vi "Script Work CS.vi"(6 "State":T1={"Worker Library Path"=path "", "Block Label"="", "Types"=[], "Selections"=[], "Icon"={"image type"=0, "image depth"=0, "image"=[], "mask"=[], "colors"=[], "Rectangle"={"left"=0, "top"=0, "right"=0, "bottom"=0}}, "Errors"={"Terminals"=[], "Generate"={"status"=FALSE, "code"=0, "source"=""}, "General"={"status"=FALSE, "code"=0, "source"=""}}, "Calculated Sizes"={"Block Width"=0, "Block Height"=0, "Half Width"=0, "Icon Top"=0, "Icon Bottom"=0, "Label Width"=0, "Half Label"=0, "Label Top"=0, "Text Width"=0, "Half Text"=0, "Text Height"=0, "Label Height"=0, "Expanded Width"=0, "Label Bottom"=0, "Expanded Top"=0, "Expanded Bottom"=0, "Expanded Height"=0, "Min Height"=0, "Max Height"=0}, "Special Terminal Indices"={"Action"=-1, "Init"=-1, "Tag"=-1, "State in"=-1, "State out"=-1, "Error"=-1, "Control"=-1}, "Terminals"=[]}, 8 "error in (no error)":errorcluster, 11 "Refs In":T13) -> (0 "error out":errorcluster, 3 "Refs":T13)   [LabVIEW 2022 SP3, in "FlexBlocks Support.lvlib"]
uses:
  FlexBlocks Support.lvlib
  SM Refs.ctl
  Flex Block/State.ctl
  Type Descriptor.ctl
  Terminal Direction.ctl
  Value Mode.ctl
  Special Terminal.ctl
  <vilib>/picture/picture.llb/imagedata.ctl
  XNode Errors.ctl
  Calculated Sizes.ctl
  Special Terminal Indices.ctl
  Terminal Status.ctl
  Terminal State.ctl
  Terminal Draw Style.ctl
  Flex Block/Flex Block.xnode
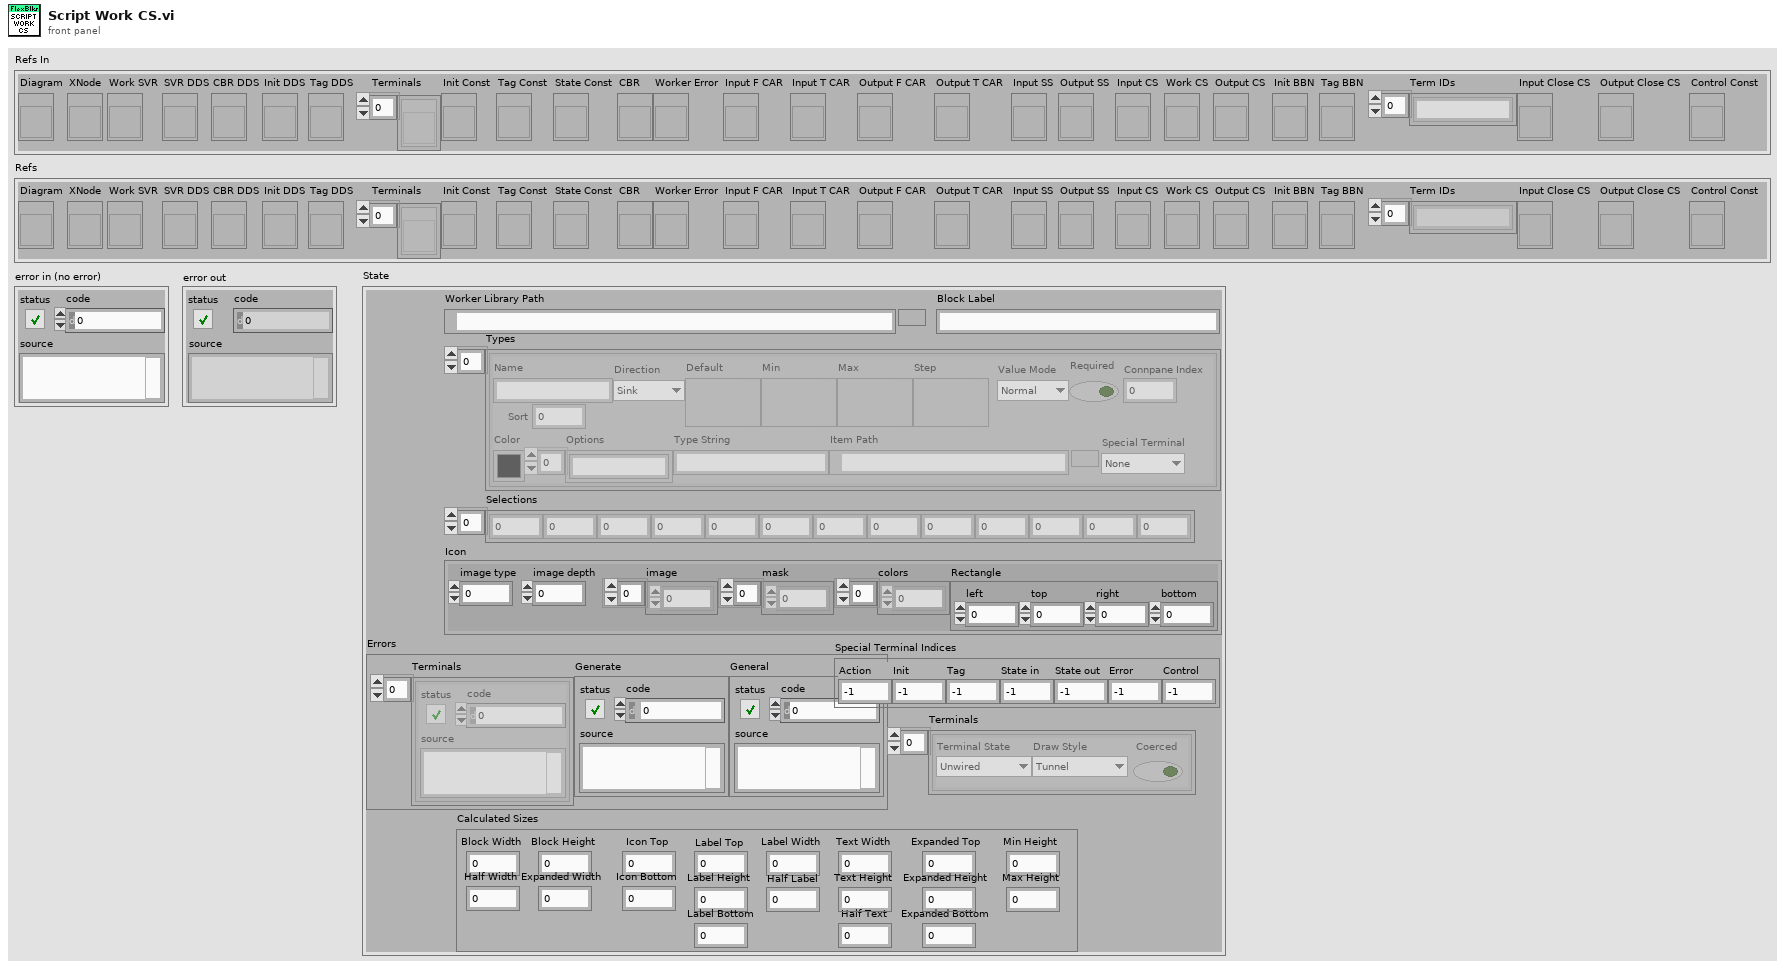
[diagram p1: front panel]
types:
  T1 = typedef "Flex Block.xnode/State.ctl" = cluster{"Worker Library Path":path, "Block Label":string, "Types":T2[], "Selections":i32[], "Icon":T6, "Errors":T7, "Calculated Sizes":T8, "Special Terminal Indices":T9, "Terminals":T10[]}
  T2 = typedef "FlexBlocks Support.lvlib/Type Descriptor.ctl" = cluster{"Name":string, "Direction":T3, "Default":variant, "Min":variant, "Max":variant, "Step":variant, "Value Mode":T4, "Color":u32, "Options":string[], "Type String":string, "Item Path":path, "Required":bool, "Connpane Index":i32, "Special Terminal":T5, "Sort":i32}
  T3 = typedef "FlexBlocks Support.lvlib/Terminal Direction.ctl" = enum16{"Sink", "Source"}
  T4 = typedef "FlexBlocks Support.lvlib/Value Mode.ctl" = enum16{"Normal", "Range", "Select"}
  T5 = typedef "FlexBlocks Support.lvlib/Special Terminal.ctl" = enum16{"None", "Action", "Init", "Tag", "State in", "State out", "Error", "Control"}
  T6 = typedef "imagedata.ctl" = cluster{"image type":i32, "image depth":i32, "image":u8[], "mask":u8[], "colors":u32[], "Rectangle":cluster{"left":i16, "top":i16, "right":i16, "bottom":i16}}
  T7 = typedef "FlexBlocks Support.lvlib/XNode Errors.ctl" = cluster{"Terminals":errorcluster[], "Generate":errorcluster, "General":errorcluster}
  T8 = typedef "FlexBlocks Support.lvlib/Calculated Sizes.ctl" = cluster{"Block Width":i32, "Block Height":i32, "Half Width":i32, "Icon Top":i32, "Icon Bottom":i32, "Label Width":i32, "Half Label":i32, "Label Top":i32, "Text Width":i32, "Half Text":i32, "Text Height":i32, "Label Height":i32, "Expanded Width":i32, "Label Bottom":i32, "Expanded Top":i32, "Expanded Bottom":i32, "Expanded Height":i32, "Min Height":i32, "Max Height":i32}
  T9 = typedef "FlexBlocks Support.lvlib/Special Terminal Indices.ctl" = cluster{"Action":i32, "Init":i32, "Tag":i32, "State in":i32, "State out":i32, "Error":i32, "Control":i32}
  T10 = typedef "FlexBlocks Support.lvlib/Terminal Status.ctl" = cluster{"Terminal State":T11, "Draw Style":T12, "Coerced":bool}
  T11 = typedef "FlexBlocks Support.lvlib/Terminal State.ctl" = enum16{"Unwired", "BadType", "BadRef", "Channel", "Value", "Control Ref"}
  T12 = typedef "FlexBlocks Support.lvlib/Terminal Draw Style.ctl" = enum16{"Tunnel", "BadType", "BadRef", "Channel", "Value", "Control Ref"}
  T13 = typedef "FlexBlocks Support.lvlib/SM Refs.ctl" = cluster{"Diagram":refnum<vi>, "XNode":refnum<vi>, "Work SVR":refnum<vi>, "SVR DDS":refnum<vi>, "CBR DDS":refnum<vi>, "Init DDS":refnum<vi>, "Tag DDS":refnum<vi>, "Terminals":refnum<vi>[], "Init Const":refnum<vi>, "Tag Const":refnum<vi>, "State Const":refnum<vi>, "CBR":refnum<vi>, "Worker Error":refnum<vi>, "Input F CAR":refnum<vi>, "Input T CAR":refnum<vi>, "Output F CAR":refnum<vi>, "Output T CAR":refnum<vi>, "Input SS":refnum<vi>, "Output SS":refnum<vi>, "Input CS":refnum<vi>, "Work CS":refnum<vi>, "Output CS":refnum<vi>, "Init BBN":refnum<vi>, "Tag BBN":refnum<vi>, "Term IDs":string[], "Input Close CS":refnum<vi>, "Output Close CS":refnum<vi>, "Control Const":refnum<vi>}
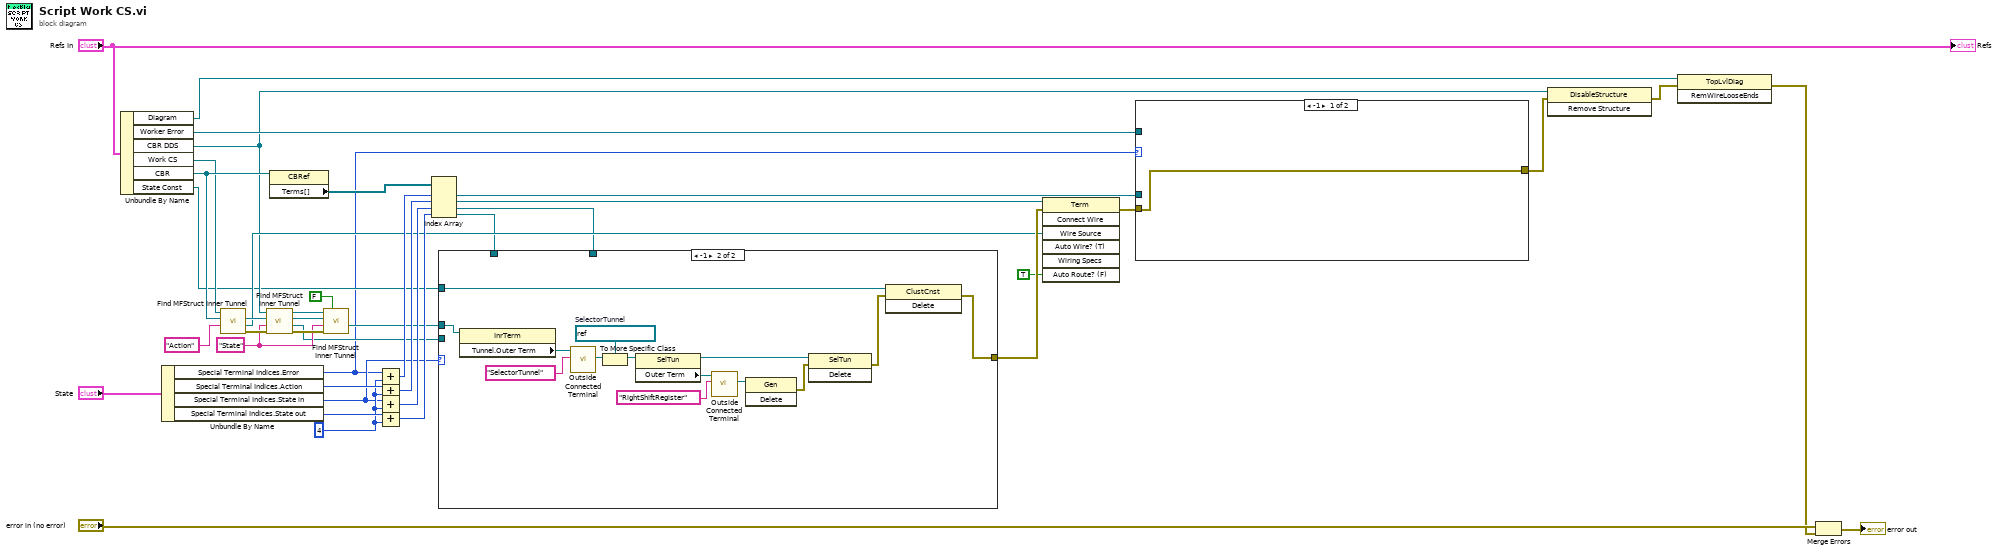
[diagram p0: block diagram]
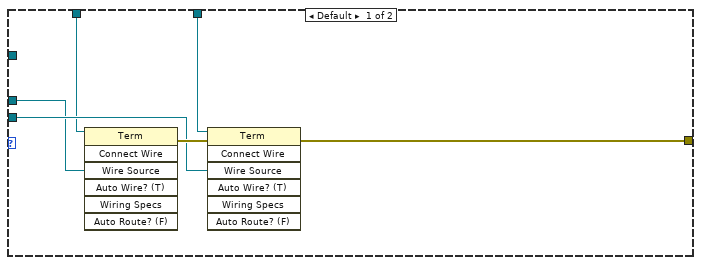
[diagram p2: hidden frame]
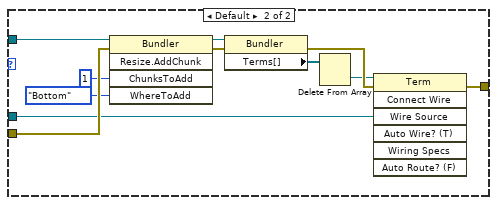
[diagram p3: hidden frame]
diagram:
  w27 = 4 ("y")
  w35 = "State" ("Tunnel Name")
  n1 = Unbundle By Name("Refs In") -> ("Diagram"=w5:refnum<vi>, "Worker Error"=w18:refnum<vi>, "CBR DDS"=w13:refnum<vi>, "Work CS"=w12:refnum<vi>, "CBR"=w20:refnum<vi>, "State Const"=w4:refnum<vi>)
  n2 = Unbundle By Name("State") -> ("Special Terminal Indices.Error"=w1:i32, "Special Terminal Indices.Action"=w28:i32, "Special Terminal Indices.State in"=w11:i32, "Special Terminal Indices.State out"=w31:i32)
  n3 = call "Find MFStruct Inner Tunnel.vi"("Tunnel Name"="Action", "Contained GObject"=w20, "MFStruct"=w12) -> ("error IO"=w39:errorcluster, "Inside Tunnel"=w19:refnum<vi>, "GObject dup"=w22:refnum<vi>)  [unwired: 5 in, 1 out]
  n4 = call "Find MFStruct Inner Tunnel.vi"("error in (no error)"=w39, "Tunnel Name"=w35, "Contained GObject"=w22, "MFStruct"=w13) -> ("error IO"=w38:errorcluster, "Inside Tunnel"=w9:refnum<vi>, "GObject dup"=w36:refnum<vi>, "MFStruct dup"=w34:refnum<vi>)  [unwired: 4 in]
  n5 = property class="CBRef"(reference=w20) -> ("Terms[]"=w32:refnum<vi>[])  [unwired: 1 in, 2 out]
  n6 = call "Find MFStruct Inner Tunnel.vi"("Source? (T)"=FALSE, "error in (no error)"=w38, "Tunnel Name"=w35, "Contained GObject"=w36, "MFStruct"=w34) -> ("Inside Tunnel"=w7:refnum<vi>)  [unwired: 3 in, 3 out]
  n7 = Add(x=w1, y=w27) -> (x+y=w25:i32)
  n8 = Add(x=w28, y=w27) -> (x+y=w26:i32)
  n9 = Add(x=w11, y=w27) -> (x+y=w30:i32)
  n10 = Add(x=w31, y=w27) -> (x+y=w29:i32)
  n11 = Index Array(array=w32, index #1=w25, index #2=w26, index #3=w30, index #4=w29) -> (element #1=w17:refnum<vi>, element #2=w24:refnum<vi>, element #3=w10:refnum<vi>, element #4=w8:refnum<vi>)
  n12 = case shown="-1" w11 {
    tunnel: w10 -> [w46 _]
    tunnel: w9 -> [w45 _]
    tunnel: w8 -> [w44 _]
    tunnel: w7 -> [w43 w61]
    tunnel: [w42 w48] -> w41
    tunnel: w4 -> [_ w50]
    frame Default {
      n13 = invoke class="Term" method="Connect Wire"(reference=w44, "Wire Source"=w43) -> (error out=w47:errorcluster)  [unwired: 5 in, 6 out]
      n14 = invoke class="Term" method="Connect Wire"(reference=w46, error in=w47, "Wire Source"=w45) -> (error out=w42:errorcluster)  [unwired: 4 in, 6 out]
    }
    frame -1 {
      w60 = refnum<vi> refnum  # SelectorTunnel
      n15 = property class="InrTerm"(reference=w61) -> ("Tunnel.Outer Term"=w58:refnum<vi>)  [unwired: 1 in, 2 out]
      n16 = call "Outside Connected Terminal.vi"("ClassType"="SelectorTunnel", "Terminal Ref In"=w58) -> ("Ref"=w52:refnum<vi>)  [unwired: 7 in, 2 out]
      n17 = To More Specific Class(target class=w60, reference=w52) -> (specific class reference=w57:refnum<vi>)  [unwired: 1 in, 1 out]
      n18 = property class="SelTun"(reference=w57) -> (reference out=w54:refnum<vi>, "Outer Term"=w56:refnum<vi>)  [unwired: 1 in, 1 out]
      n19 = call "Outside Connected Terminal.vi"("ClassType"="RightShiftRegister", "Terminal Ref In"=w56) -> ("Ref"=w51:refnum<vi>)  [unwired: 7 in, 2 out]
      n20 = invoke class="Gen" method="Delete"(reference=w51) -> (error out=w53:errorcluster)  [unwired: 2 in, 2 out]
      n21 = invoke class="SelTun" method="Delete"(reference=w54, error in=w53) -> (error out=w49:errorcluster)  [unwired: 1 in, 2 out]
      n22 = invoke class="ClustCnst" method="Delete"(reference=w50, error in=w49) -> (error out=w48:errorcluster)  [unwired: 1 in, 2 out]
    }
  }
  n23 = invoke class="Term" method="Connect Wire"(reference=w24, error in=w41, "Wire Source"=w19, "Auto Route? (F)"=TRUE) -> (error out=w40:errorcluster)  [unwired: 3 in, 6 out]
  n24 = case shown="-1" w1 {
    tunnel: w40 -> [w62 w72]
    tunnel: w18 -> [_ w71]
    tunnel: w17 -> [_ w64]
    tunnel: [w62 w63] -> w14
    frame -1 {
    }
    frame Default {
      n25 = invoke class="Bundler" method="Resize.AddChunk"(reference=w71, error in=w72, "ChunksToAdd"=u8 1 ("Chunks To Add"), "WhereToAdd"=enum8{"Bottom", "Top"}."Bottom" ("Where To Add")) -> (reference out=w68:refnum<vi>, error out=w67:errorcluster)  [unwired: 1 in, 3 out]
      n26 = property class="Bundler"(reference=w68, error in=w67) -> (error out=w73:errorcluster, "Terms[]"=w66:refnum<vi>[])  [unwired: 1 out]
      n27 = Delete From Array(array=w66) -> (deleted portion=w65:refnum<vi>)  [unwired: 2 in, 1 out]
      n28 = invoke class="Term" method="Connect Wire"(reference=w65, error in=w73, "Wire Source"=w64) -> (error out=w63:errorcluster)  [unwired: 4 in, 6 out]
    }
  }
  n29 = invoke class="DisableStructure" method="Remove Structure"(reference=w13, error in=w14) -> (error out=w3:errorcluster)  [unwired: 1 in, 2 out]
  n30 = invoke class="TopLvlDiag" method="RemWireLooseEnds"(reference=w5, error in=w3) -> (error out=w2:errorcluster)  [unwired: 1 in, 2 out]
  n31 = Merge Errors("error in (no error)", w2) -> (→"error out":errorcluster)
  "Refs" <- "Refs In"
